vi "gu_is_text_utf16.vi"(8 "error in":errorcluster, 11 "String":string) -> (0 "error out":errorcluster, 3 "Encoding":T1)   [LabVIEW 2020, in "G-Unicode.lvlib"]
uses:
  G-Unicode.lvlib
  Unicode/Controls/String Encoding.ctl
  lib/g_unicode_32.dll
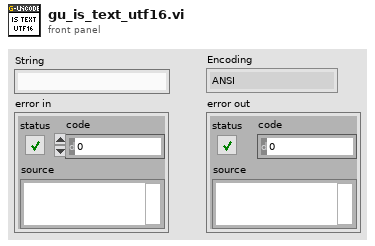
[diagram p1: front panel]
types:
  T1 = typedef "G-Unicode.lvlib/String Encoding.ctl" = enum16{"ANSI", "UTF-8", "UTF-16LE", "UTF-16BE", "Unknown"}
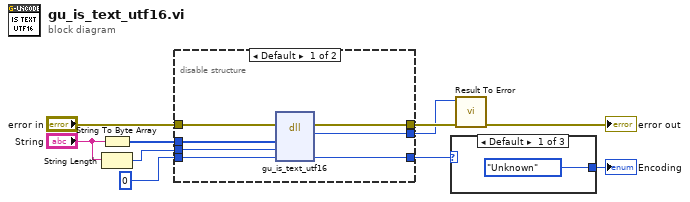
[diagram p0: block diagram]
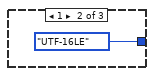
[diagram p2: hidden frame]
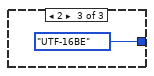
[diagram p3: hidden frame]
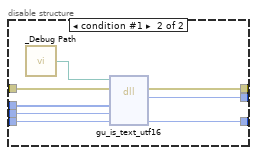
[diagram p4: hidden frame]
diagram:
  n1 = String To Byte Array(string="String") -> (unsigned byte array=w9:u8[])
  n2 = String Length(string="String") -> (length=w7:i32)
  n3 = disable-structure shown="Default" {
    disable-tunnel: w9 -> [w15 w23]
    disable-tunnel: [w12 w19] -> w6
    disable-tunnel: "error in" -> [w17 w25]
    disable-tunnel: [w16 w24] -> w3
    disable-tunnel: w7 -> [w14 w22]
    disable-tunnel: 0 ("utf16") -> [w13 w20]
    disable-tunnel: [w11 w18] -> w1
    frame condition #0 (active) {
      n4 = dll-call lib="C:/github/dataflowg/g-unicode/src/LabVIEW/G-Unicode/lib/g_unicode_*.*" fn="gu_is_text_utf16"(error in=w17, "buf"=w15, "size"=w14, "is_utf16"=w13) -> (error out=w16:errorcluster, "result"=w11:i32, "is_utf16"=w12:i32)  [unwired: 4 in, 1 out]
    }
    frame condition #1 {
      n5 = call "_Debug Path.vi"() -> ("Debug Path"=w21:path)
      n6 = dll-call lib="?" fn="gu_is_text_utf16"(path in=w21, error in=w25, "buf"=w23, "size"=w22, "is_utf16"=w20) -> (error out=w24:errorcluster, "result"=w18:i32, "is_utf16"=w19:i32)  [unwired: 3 in, 1 out]
    }
  }
  n7 = case shown="Default" w6 {
    tunnel: [String_Encoding."Unknown" ("Encoding") String_Encoding."UTF-16LE" ("Encoding") String_Encoding."UTF-16BE" ("Encoding")] -> w5
    frame Default {
    }
    frame 1 {
    }
    frame 2 {
    }
  }
  "Encoding" <- w5
  n8 = call "Result To Error.vi"("error in (no error)"=w3, "Result Code"=w1) -> ("error out"=→"error out":errorcluster)  [unwired: 9 in]
